vi "Select Role.vi"(8 "error in (no error)":errorcluster, 10 "Role":string, 11 "Role Manager in":refnum<class "Role Manager.lvclass">) -> (0 "error out":errorcluster, 3 "Role Manager out":refnum<class "Role Manager.lvclass">)   [LabVIEW 2020, in "Volatus.lvlib" / "Role Manager.lvclass"]
uses:
  Role Manager.lvclass
  C:/dev/lv20CE/relink/lv-volatus/Volatus/Module/Module.lvclass
  Role Manager.lvclass/Role Manager.ctl
  Module/Module.lvclass/Module.ctl
  Roles API/Roles API.lvclass
  Module/Module.lvclass
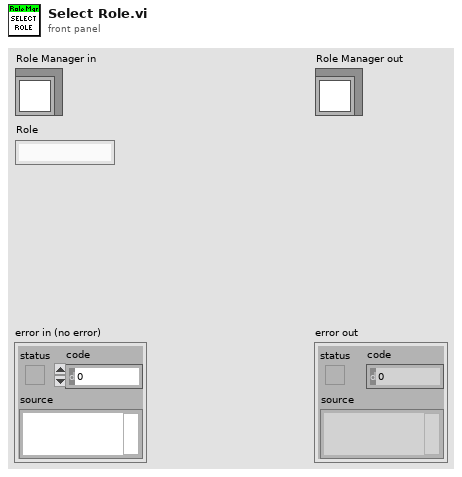
[diagram p1: front panel]
types:
  T1 = typedef "Volatus.lvlib/Role Manager.lvclass/Role Info.ctl" = cluster{"Name":string, "Hidden":bool, "Effective Roles":set{string}}
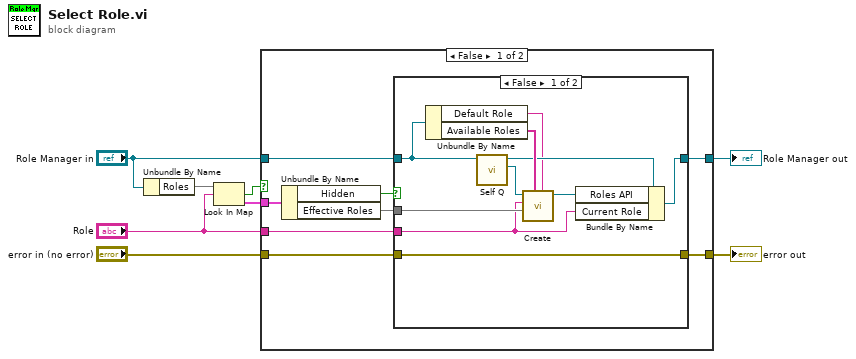
[diagram p0: block diagram]
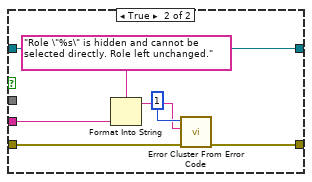
[diagram p2: hidden frame]
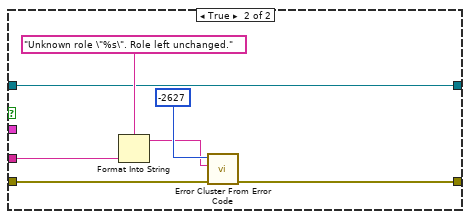
[diagram p3: hidden frame]
diagram:
  n1 = Unbundle By Name("Role Manager in") -> ("Roles"=w8:map{string, T1})
  n2 = Look In Map(map=w8, key="Role") -> (key not found?=w6:bool, value=w5:T1)  [unwired: 1 in]
  n3 = case shown="False" w6 {
    tunnel: "Role Manager in" -> [w14 w34]
    tunnel: w5 -> [w16 _]
    tunnel: "Role" -> [w13 w40]
    tunnel: [w11 w36] -> w2
    tunnel: "error in (no error)" -> [w12 w35]
    tunnel: [w9 w34] -> w1
    frame False {
      n4 = Unbundle By Name(w16) -> ("Hidden"=w15:bool, "Effective Roles"=w10:set{string})
      n5 = case shown="False" w15 {
        tunnel: w14 -> [w25 w33]
        tunnel: w13 -> [w20 w32]
        tunnel: w12 -> [w18 w30]
        tunnel: [w18 w27] -> w11
        tunnel: w10 -> [w23 _]
        tunnel: [w19 w33] -> w9
        frame False {
          n6 = Unbundle By Name(w25) -> ("Default Role"=w17:string, "Available Roles"=w26:string[])
          n7 = call "Self Q.vi"("Module in"=w25) -> ("Self Q"=w24:refnum<class "MessageQ.lvclass">, "Module out"=w22:refnum<class "Role Manager.lvclass">)  [unwired: 9 in]
          n8 = call "Create.vi"("Default Role"=w17, "Available"=w26, "Effective Roles"=w23, "Current Role"=w20, "Manager"=w24) -> ("Roles API out"=w21:refnum<class "Roles API.lvclass">)  [unwired: 5 in, 1 out]
          n9 = Bundle By Name(cluster=w22, "Roles API"=w21, "Current Role"=w20) -> (w19:refnum<class "Role Manager.lvclass">)
        }
        frame True {
          n10 = Format Into String(format string="Role \"%s\" is hidden and cannot be selected directly. Role left unchanged.", w32) -> (resulting string=w28:string)  [unwired: 2 in, 1 out]
          n11 = call <vilib>:"Error Cluster From Error Code.vi"("error in (no error)"=w30, "error message (\"\")"=w28, "error code (0)"=1) -> ("error out"=w27:errorcluster)  [unwired: 6 in]
        }
      }
    }
    frame True {
      n12 = Format Into String(format string="Unknown role \"%s\". Role left unchanged.", w40) -> (resulting string=w37:string)  [unwired: 2 in, 1 out]
      n13 = call <vilib>:"Error Cluster From Error Code.vi"("error in (no error)"=w35, "error message (\"\")"=w37, "error code (0)"=-2627) -> ("error out"=w36:errorcluster)  [unwired: 6 in]
    }
  }
  "error out" <- w2
  "Role Manager out" <- w1
